vi "Create_Object.vi"(8 "error in (no error)":errorcluster, 9 "Block Diagram in":T1, 10 "owner refnum":variant, 11 "SubVI in":refnum<class "SubVI.lvclass">) -> (0 "error out":errorcluster, 1 "Block Diagram Out":T1, 3 "SubVI out":refnum<class "SubVI.lvclass">)   [LabVIEW 2025, in "SubVI.lvclass"]
uses:
  SubVI.lvclass
  C:/Users/mrjak/Documents/GitHub/LVGPT/LabVIEW/VIs/Classes/Node/Node.lvclass
  Controls/bd.ctl
  Node.lvclass
  Controls/wire.ctl
  Controls/Terminal.ctl
  Node.lvclass/Node.ctl
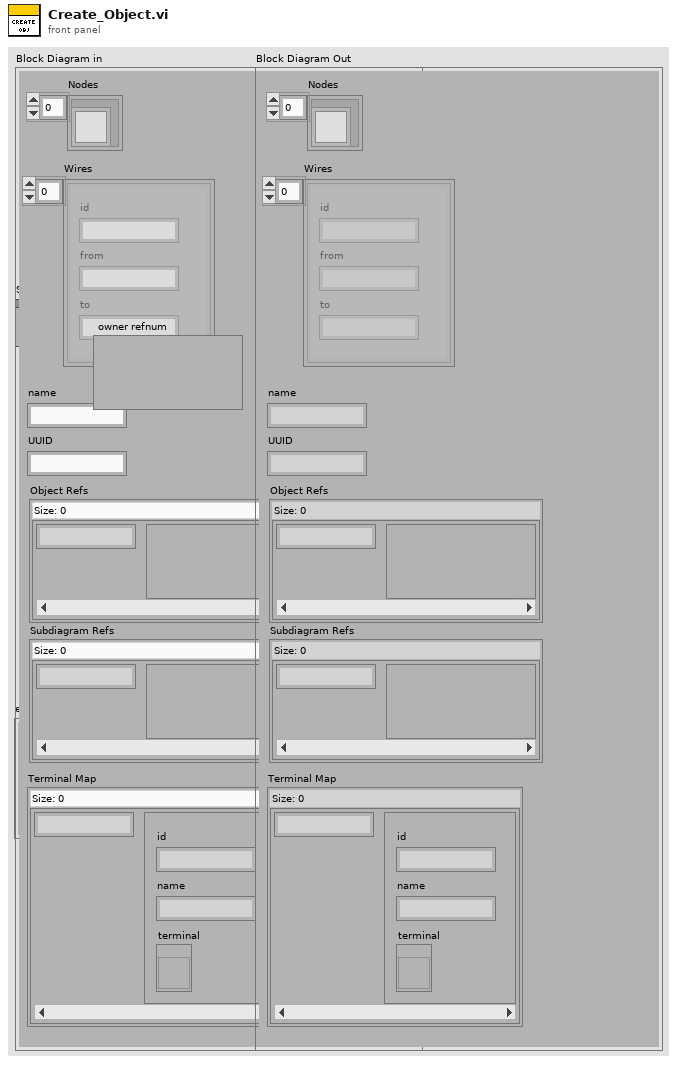
[diagram p1: front panel]
types:
  T1 = typedef "bd.ctl" = cluster{"Nodes":refnum<class "Node.lvclass">[], "Wires":T2[], "name":string, "UUID":string, "Object Refs":map{string, variant}, "Subdiagram Refs":map{string, variant}, "Terminal Map":map{string, T3}}
  T2 = typedef "wire.ctl" = cluster{"id":string, "from":string, "to":string}
  T3 = typedef "Terminal.ctl" = cluster{"id":string, "name":string, "terminal":refnum<vi>}
  T4 = typedef "LVPointTypeDef.ctl" = cluster{"Horizontal":i16, "Vertical":i16}
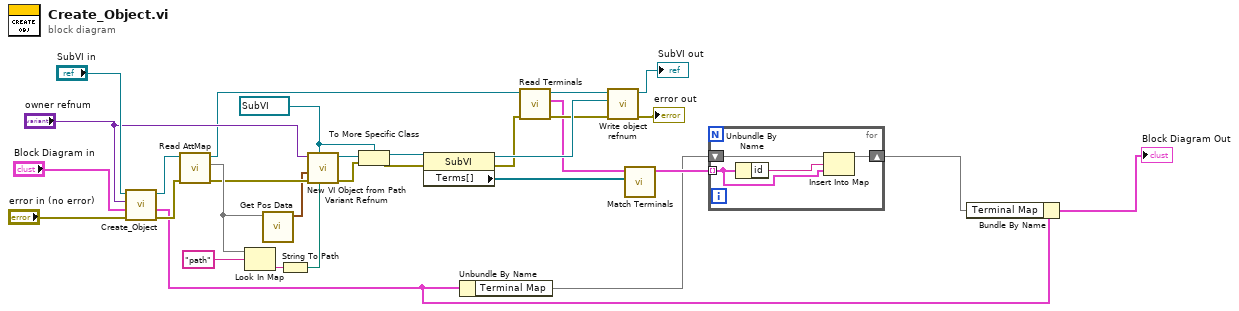
[diagram p0: block diagram]
diagram:
  w17 = refnum<vi> refnum ("vi object class")
  n1 = call-parent "Create_Object.vi"("error in (no error)"="error in (no error)", "Block Diagram in"="Block Diagram in", "owner refnum"="owner refnum", "Node in"="SubVI in") -> ("error out"=w28:errorcluster, "Block Diagram Out"=w3:T1, "Node out"=w27:refnum<class "SubVI.lvclass">)  [unwired: 5 in]
  n2 = call "Read AttMap.vi"("error in (no error)"=w28, "Node in"=w27) -> ("error out"=w24:errorcluster, "AttMap"=w25:map{string, string}, "Node out"=w11:refnum<class "SubVI.lvclass">)  [unwired: 7 in]
  n3 = Look In Map(map=w25, key="path") -> (value=w21:string)  [unwired: 1 in, 1 out]
  n4 = call "Get Pos Data.vi"("AttMap"=w25) -> ("Position"=w22:T4)  [unwired: 10 in]
  n5 = String To Path(string=w21) -> (path=w20:path)
  n6 = call "New VI Object from Path Variant Refnum.vi"("path"=w20, "vi object class"=w17, "error in (no error)"=w24, "location"=w22, "owner refnum"="owner refnum") -> ("error out"=w19:errorcluster, "object refnum"=w18:refnum<vi>)  [unwired: 5 in]
  n7 = To More Specific Class(target class=w17, reference=w18, error in=w19) -> (specific class reference=w13:refnum<vi>, error out=w12:errorcluster)
  n8 = property class="SubVI"(reference=w13, error in=w12) -> (reference out=w14:refnum<vi>, error out=w7:errorcluster, "Terms[]"=w16:refnum<vi>[])
  n9 = Unbundle By Name(w3) -> ("Terminal Map"=w4:map{string, T3})
  n10 = call "Read Terminals.vi"("error in (no error)"=w7, "Node in"=w11) -> ("error out"=w6:errorcluster, "Terminals"=w5:T3[], "Node out"=w8:refnum<class "SubVI.lvclass">)  [unwired: 7 in]
  n11 = call-dynamic "Write object refnum.vi"("error in (no error)"=w6, "object refnum"=w14, "Node in"=w8) -> ("error out"=→"error out":errorcluster, "Node out"=→"SubVI out":refnum<class "SubVI.lvclass">)  [unwired: 7 in]
  n12 = call "Match Terminals.vi"("Terms[]"=w16, "Terminals"=w5) -> ("Terminals Out"=w15:T3[])  [unwired: 9 in]
  n13 = for {
    shift-right: [w34] -> w2
    shift-left: w4 -> [w35]
    tunnel: w15 -> [w33] mode=indexing
    n14 = Unbundle By Name(w33) -> ("id"=w32:string)
    n15 = Insert Into Map(map in=w35, key=w32, value=w33) -> (map out=w34:map{string, T3})  [unwired: 2 out]
  }
  n16 = Bundle By Name(cluster=w3, "Terminal Map"=w2) -> (→"Block Diagram Out":T1)
